vi "DAQmx Channel Init Error.vi"(8 "error in":errorcluster) -> (0 "error out":errorcluster, 3 "channel init error?":bool)   [LabVIEW 2011, in "Mass Flow Controller.lvclass"]
uses:
  Mass Flow Controller.lvclass
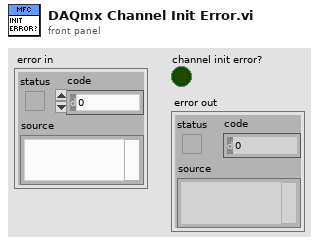
[diagram p1: front panel]
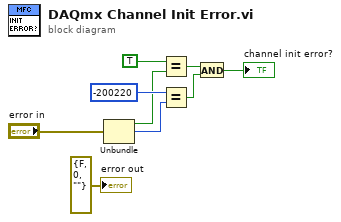
[diagram p0: block diagram]
diagram:
  n1 = Unbundle("error in") -> ("status"=w4:bool, "code"=w3:i32)  [unwired: 1 out]
  n2 = Equal?(x=TRUE ("status"), y=w4) -> (x = y?=w6:bool)
  n3 = Equal?(x=-200220 ("code"), y=w3) -> (x = y?=w7:bool)
  n4 = And(x=w6, y=w7) -> (x .and. y?=→"channel init error?":bool)
  "error out" <- errorcluster {"status"=FALSE, "code"=0, "source"=""} ("error out")
